vi "Module Cleanup.vi"(8 "error in (no error)":errorcluster, 11 "DAQmxDO in":refnum<class "DAQmxDO.lvclass">) -> (0 "error out":errorcluster, 3 "DAQmxDO out":refnum<class "DAQmxDO.lvclass">)   [LabVIEW 2020, in "VolatusDAQ.lvlib" / "DAQmxDO.lvclass"]
uses:
  DAQmxDO.lvclass
  DAQmxDO.lvclass/DAQmxDO.ctl
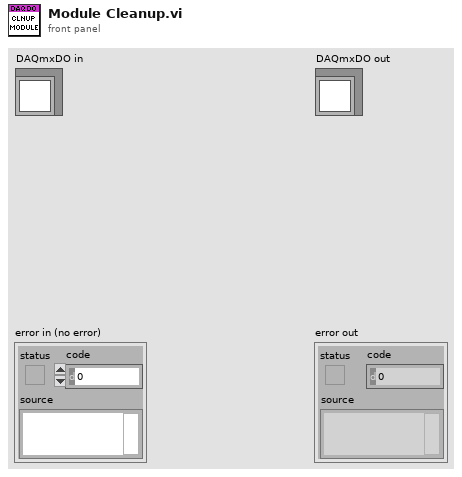
[diagram p1: front panel]
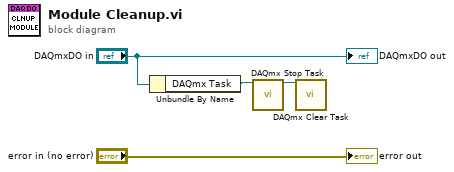
[diagram p0: block diagram]
diagram:
  n1 = Unbundle By Name("DAQmxDO in") -> ("DAQmx Task"=w3:refnum<k21>)
  n2 = call <vilib>:"DAQmx Stop Task.vi"("task/channels in"=w3) -> ("task out"=w2:refnum<k21>)  [unwired: 13 in, 1 out]
  n3 = call <vilib>:"DAQmx Clear Task.vi"("task in"=w2) -> ()  [unwired: 14 in, 1 out]
  "error out" <- "error in (no error)"
  "DAQmxDO out" <- "DAQmxDO in"
